vi "Relax_freq_2024.vi"(2 "H2O molar fraction":dbl format="%_6f", 3 "Pressure [Pa]":dbl, 4 "Temperature [K]":dbl format="%.4g") -> (0 "Relax freq N2":dbl, 1 "Relax freq O2":dbl)   [LabVIEW 2016]
panel:
  # "Hz"
  # "Hz"
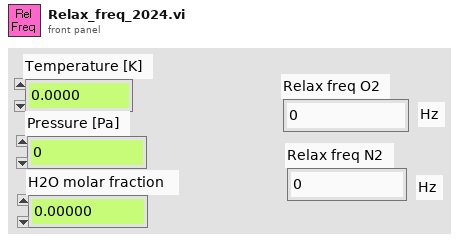
[diagram p1: front panel]
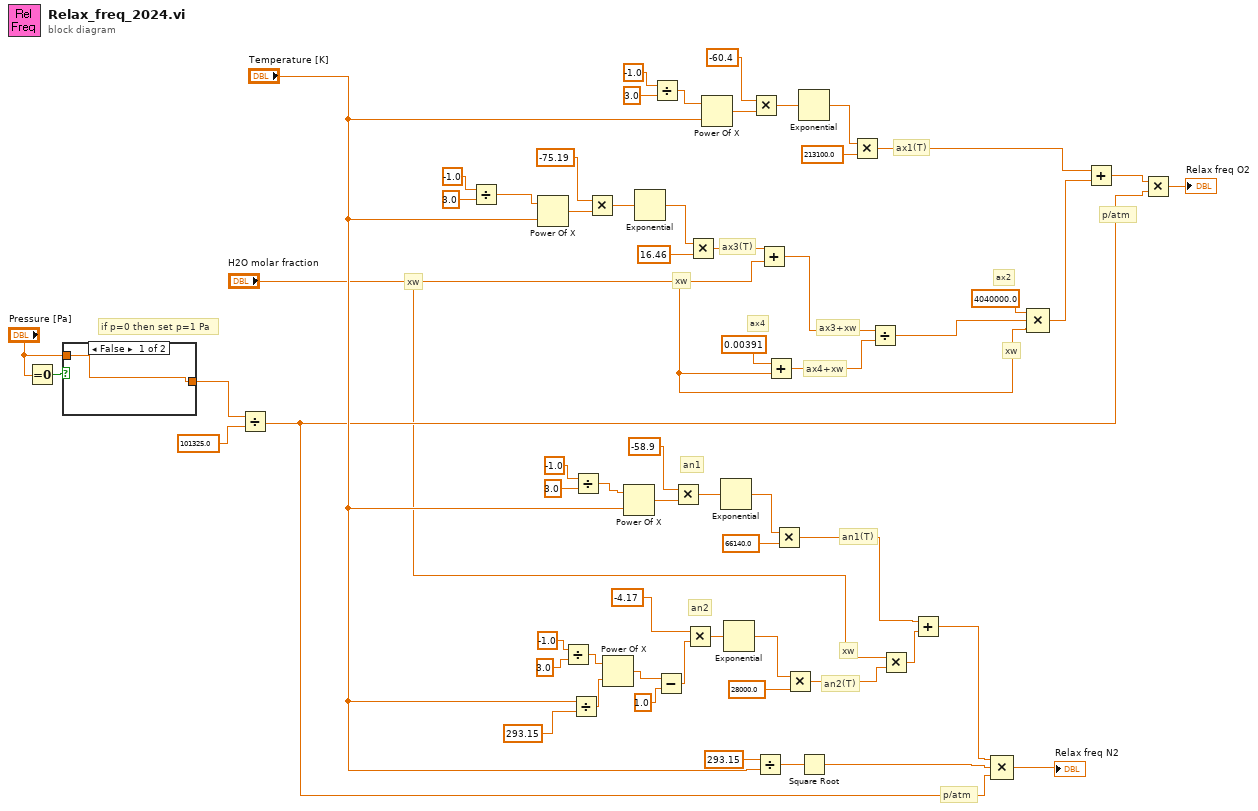
[diagram p0: block diagram]
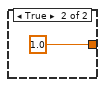
[diagram p2: hidden frame]
diagram:
  # "an1(T)"
  # "an2(T)"
  # "xw"
  # "xw"
  # "p/atm"
  # "p/atm"
  # "ax4+xw"
  # "ax3+xw"
  # "xw"
  # "xw"
  # "ax4"
  # "ax2"
  # "if p=0 then set p=1 Pa"
  # "an2"
  # "an1"
  # "ax3(T)"
  # "ax1(T)"
  n1 = Equal To 0?(x="Pressure [Pa]") -> (x = 0?=w4:bool)
  n2 = case shown="False" w4 {
    tunnel: [w62 1.0] -> w5
    tunnel: "Pressure [Pa]" -> [w62 _]
    frame False {
    }
    frame True {
    }
  }
  n3 = Divide(x=w5, y=101325.0) -> (x/y=w16:dbl)
  n4 = Divide(x=-1.0, y=3.0) -> (x/y=w9:dbl)
  n5 = Power Of X(1:"Temperature [K]", 2:w9) -> (0:w51:dbl)
  n6 = Divide(x=-1.0 ("y"), y=3.0) -> (x/y=w28:dbl)
  n7 = Divide(x="Temperature [K]", y=293.15) -> (x/y=w31:dbl)
  n8 = Divide(x=-1.0, y=3.0) -> (x/y=w6:dbl)
  n9 = Multiply(x=-75.19, y=w51) -> (x*y=w53:dbl)
  n10 = Power Of X(1:w31, 2:w28) -> (0:w27:dbl)
  n11 = Power Of X(1:"Temperature [K]", 2:w6) -> (0:w37:dbl)
  n12 = Exponential(1:w53) -> (0:w54:dbl)
  n13 = Divide(x=-1.0, y=3.0) -> (x/y=w14:dbl)
  n14 = Subtract(x=w27, y=1.0) -> (x-y=w25:dbl)
  n15 = Multiply(x=-58.9, y=w37) -> (x*y=w39:dbl)
  n16 = Multiply(x=-4.17, y=w25) -> (x*y=w34:dbl)
  n17 = Multiply(x=w54, y=16.46) -> (x*y=w48:dbl)
  n18 = Power Of X(1:"Temperature [K]", 2:w14) -> (0:w56:dbl)
  n19 = Exponential(1:w39) -> (0:w40:dbl)
  n20 = Exponential(1:w34) -> (0:w35:dbl)
  n21 = Multiply(x=-60.4, y=w56) -> (x*y=w58:dbl)
  n22 = Divide(x=293.15, y="Temperature [K]") -> (x/y=w22:dbl)
  n23 = Add(x=w48, y="H2O molar fraction") -> (x+y=w47:dbl)
  n24 = Add(x=0.00391, y="H2O molar fraction") -> (x+y=w46:dbl)
  n25 = Multiply(x=w40, y=66140.0) -> (x*y=w21:dbl)
  n26 = Multiply(x=w35, y=28000.0) -> (x*y=w20:dbl)
  n27 = Exponential(1:w58) -> (0:w59:dbl)
  n28 = Square Root(x=w22) -> (sqrt(x)=w17:dbl)
  n29 = Multiply(x=w59, y=213100.0) -> (x*y=w50:dbl)
  n30 = Divide(x=w47, y=w46) -> (x/y=w1:dbl)
  n31 = Multiply(x="H2O molar fraction", y=w20) -> (x*y=w19:dbl)
  n32 = Add(x=w21, y=w19) -> (x+y=w18:dbl)
  n33 = Compound Arithmetic op=MULTIPLY(w18, w17, w16) -> (→"Relax freq N2":dbl)
  n34 = Compound Arithmetic op=MULTIPLY(4040000.0 ("value"), w1, "H2O molar fraction") -> (w44:dbl)
  n35 = Add(x=w50, y=w44) -> (x+y=w43:dbl)
  n36 = Multiply(x=w43, y=w16) -> (x*y=→"Relax freq O2":dbl)
